vi "Pitch and Roll (SubVI).vi"(0 "Vertical Speed":sgl, 4 "yaw":dbl, 5 "Vertical movement":bool, 6 "pitch":dbl, 7 "roll":dbl, 8 "pitch offset":dbl=0.15 format="%#_13g", 9 "roll adjust":dbl=1.5 format="%#_13g") -> (3 "Control Cluster out":T1 {"Yaw Speed" scale=-1.0..1.0; "Vertical Speed" scale=-1.0..1.0; "Pitch" scale=-1.0..1.0; "Roll" scale=-1.0..1.0})   [LabVIEW 2014]
uses:
  Resources/Others/Control cluster.ctl
panel:
  in  "vertical speed offset":sgl
  in  "yaw adjust":dbl=2.0
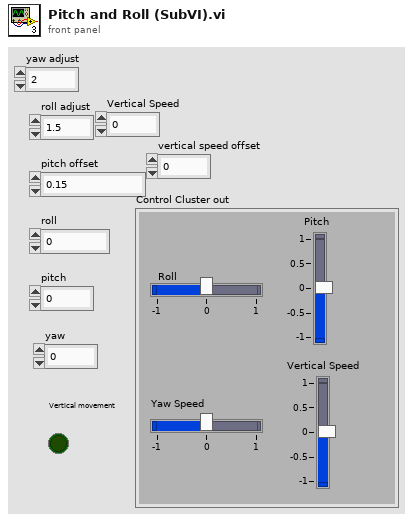
[diagram p1: front panel]
types:
  T1 = typedef "Control cluster.ctl" = cluster{"Roll":sgl, "Pitch":sgl, "Vertical Speed":sgl, "Yaw Speed":sgl}
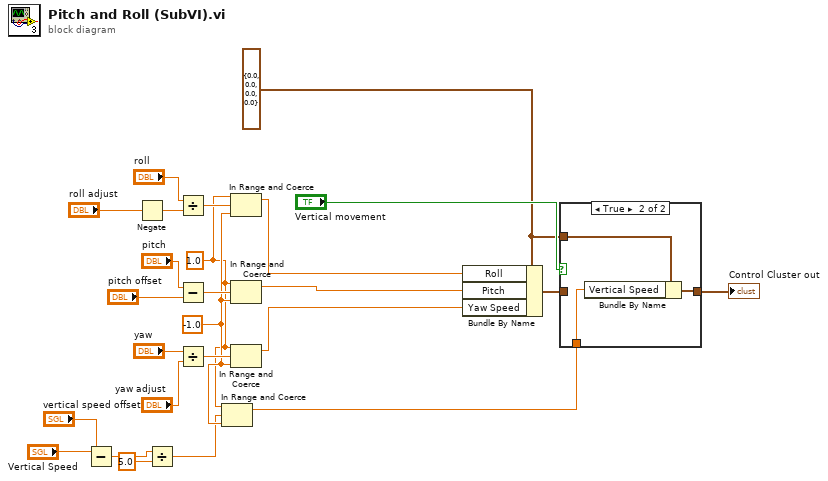
[diagram p0: block diagram]
diagram:
  w12 = -1.0 ("lower limit")
  w11 = 1.0 ("upper limit")
  w2 = T1 {"Roll"=0.0, "Pitch"=0.0, "Vertical Speed"=0.0, "Yaw Speed"=0.0} ("Control Cluster out")
  n1 = Subtract(x="Vertical Speed", y="vertical speed offset") -> (x-y=w8:sgl)
  n2 = Negate(x="roll adjust") -> (-x=w21:dbl)
  n3 = Divide(x=w8, y=sgl 5.0) -> (x/y=w7:sgl)
  n4 = Divide(x="roll", y=w21) -> (x/y=w22:dbl)
  n5 = Subtract(x="pitch", y="pitch offset") -> (x-y=w23:dbl)
  n6 = Divide(x="yaw", y="yaw adjust") -> (x/y=w14:dbl)
  n7 = In Range and Coerce(upper limit=w11, x=w7, lower limit=w12) -> (coerced(x)=w1:dbl)  [unwired: 1 out]
  n8 = In Range and Coerce(upper limit=w11, x=w22, lower limit=w12) -> (coerced(x)=w25:dbl)  [unwired: 1 out]
  n9 = In Range and Coerce(upper limit=w11, x=w23, lower limit=w12) -> (coerced(x)=w24:dbl)  [unwired: 1 out]
  n10 = In Range and Coerce(upper limit=w11, x=w14, lower limit=w12) -> (coerced(x)=w16:dbl)  [unwired: 1 out]
  n11 = Bundle By Name(cluster=w2, "Roll"=w25, "Pitch"=w24, "Yaw Speed"=w16) -> (w4:T1)
  n12 = case shown="True" "Vertical movement" {
    tunnel: w4 -> [w26 _]
    tunnel: [w26 w29] -> w3
    tunnel: w2 -> [_ w28]
    tunnel: w1 -> [_ w27]
    frame False {
    }
    frame True {
      n13 = Bundle By Name(cluster=w28, "Vertical Speed"=w27) -> (w29:T1)
    }
  }
  "Control Cluster out" <- w3
